vi "ManualArm Pneumatics.vi"   [LabVIEW 2013]
doc: "Run the pneumatics when in joystick mode"
uses:
  Team Code/Robot Global Data.vi
types:
  T1 = typedef "Gamepad.ctl" = cluster{"Buttons":T2, "Axes":cluster{"axis 1 (x)":dbl, "axis 2 (y)":dbl, "axis 3 (throttle)":dbl, "axis 4":dbl, "axis 5":dbl, "axis 6":dbl}}
  T2 = typedef "WPI_JoystickButtonState.ctl" = cluster{"Button 1":bool, "Button 2":bool, "Button 3":bool, "Button 4":bool, "Button 5":bool, "Button 6":bool, "Button 7":bool, "Button 8":bool, "Button 9":bool, "Button 10":bool, "Button 11":bool, "Button 12":bool}
  T3 = typedef "Arm Joystick.ctl" = cluster{"Buttons":T2, "Axes":cluster{"axis 1 (x)":dbl, "axis 2 (y)":dbl, "axis 3 (throttle)":dbl, "axis 4":dbl, "axis 5":dbl, "axis 6":dbl}}
  T4 = typedef "Right Drive Joystick.ctl" = cluster{"Buttons":T2, "Axes":cluster{"axis 1 (x)":dbl, "axis 2 (y)":dbl, "axis 3 (throttle)":dbl, "axis 4":dbl, "axis 5":dbl, "axis 6":dbl}}
  T5 = typedef "Left Drive Joystick.ctl" = cluster{"Buttons":T2, "Axes":cluster{"axis 1 (x)":dbl, "axis 2 (y)":dbl, "axis 3 (throttle)":dbl, "axis 4":dbl, "axis 5":dbl, "axis 6":dbl}}
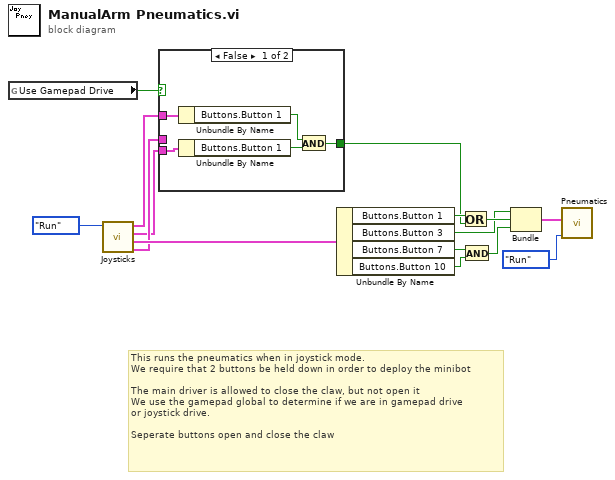
[diagram p0: block diagram]
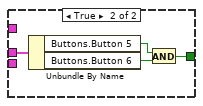
[diagram p2: hidden frame]
diagram:
  # "This runs the pneumatics when in joystick mode.\nWe require that 2 buttons be held down in order to deploy the minibot\n\nThe main driver is allowed to close the claw, but not open it\nWe use the gamepad global to determine if we are in gamepad drive\nor joystick drive.\n\nSeperate buttons open and close the claw"
  n1 = global read "Robot Global Data.vi" "Use Gamepad Drive"() -> (w5:bool)
  n2 = call "Joysticks.vi"("Mode"=enum16{"Init", "Run", "End"}."Run") -> ("GamePad"=w4:T1, "Arm Joystick"=w10:T3, "Right Driving Joystick Values"=w2:T4, "Left Driving Joystick Values"=w3:T5)  [unwired: 5 out]
  n3 = case shown="False" w5 {
    tunnel: w2 -> [w20 _]
    tunnel: w3 -> [w19 _]
    tunnel: [w18 w21] -> w1
    tunnel: w4 -> [_ w22]
    frame False {
      n4 = Unbundle By Name(w19) -> ("Buttons.Button 1"=w17:bool)
      n5 = Unbundle By Name(w20) -> ("Buttons.Button 1"=w16:bool)
      n6 = And(x=w17, y=w16) -> (x .and. y?=w18:bool)
    }
    frame True {
      n7 = Unbundle By Name(w22) -> ("Buttons.Button 5"=w24:bool, "Buttons.Button 6"=w23:bool)
      n8 = And(x=w24, y=w23) -> (x .and. y?=w21:bool)
    }
  }
  n9 = Unbundle By Name(w10) -> ("Buttons.Button 1"=w14:bool, "Buttons.Button 3"=w6:bool, "Buttons.Button 7"=w12:bool, "Buttons.Button 10"=w11:bool)
  n10 = Or(x=w14, y=w1) -> (x .or. y?=w8:bool)
  n11 = And(x=w12, y=w11) -> (x .and. y?=w9:bool)
  n12 = Bundle("Button 3"=w6, w8, w9) -> (w7:cluster{"Button 3":bool, bool, bool})  [unwired: 1 out]
  n13 = call "Pneumatics.vi"("Mode"=enum16{"Init", "Run", "End"}."Run", "Inputs"=w7) -> ()  [unwired: 3 in, 7 out]
